vi "GetFitValues.vi"(8 "error in (no error)":errorcluster, 11 "Mean Fit in":refnum<class "Mean Fit.lvclass">) -> (0 "error out":errorcluster, 2 "Mean Fit":T1, 3 "Mean Fit out":refnum<class "Mean Fit.lvclass">)   [LabVIEW 2013, in "Mean Fit.lvclass"]
uses:
  Mean Fit.lvclass
  Mean Fit.lvclass/Mean Fit.ctl
panel:
  # "Stimulus"
  # "Response"
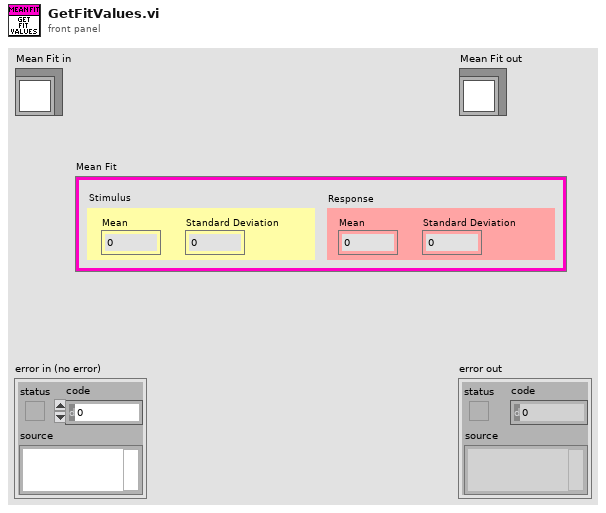
[diagram p1: front panel]
types:
  T1 = cluster{"Respopnse Mean":dbl, "Response SD":dbl, "Stimulus Mean":dbl, "Stimulus SD":dbl}
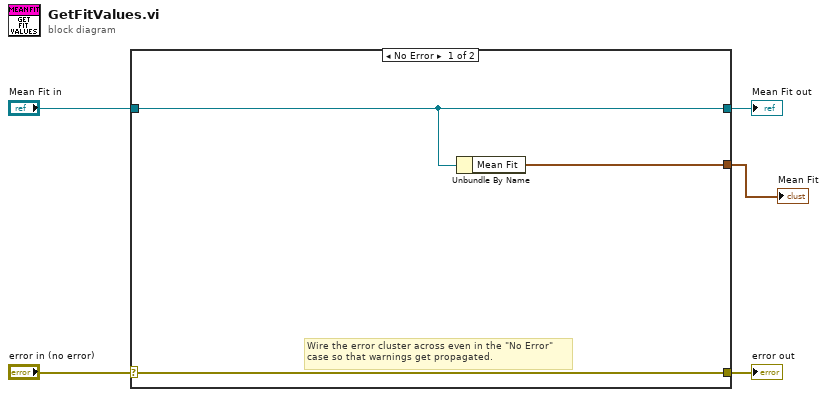
[diagram p0: block diagram]
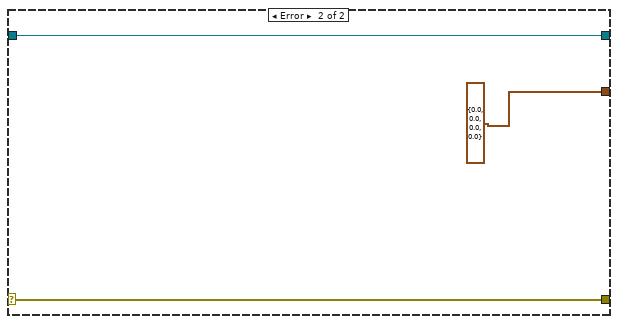
[diagram p2: hidden frame]
diagram:
  n1 = case shown="No Error" "error in (no error)" {
    selector: "error in (no error)" -> [w8 w11]
    tunnel: [w8 w11] -> w4
    tunnel: [w7 w10] -> w2
    tunnel: "Mean Fit in" -> [w7 w10]
    tunnel: [w6 T1 {"Respopnse Mean"=0.0, "Response SD"=0.0, "Stimulus Mean"=0.0, "Stimulus SD"=0.0} ("Mean Fit")] -> w1
    frame No Error {
      # "Wire the error cluster across even in the \"No Error\"\ncase so that warnings get propagated."
      n2 = Unbundle By Name(w7) -> ("Mean Fit"=w6:T1)
    }
    frame Error {
    }
  }
  "error out" <- w4
  "Mean Fit out" <- w2
  "Mean Fit" <- w1
